vi "Check if string is integer.vi"(8 "error in (no error)":errorcluster, 11 "string in":string) -> (0 "error out":errorcluster, 2 "T = string contains an integer":bool, 3 "string out (duplicate)":string)   [LabVIEW 2021, in "Numeric Utilities.lvlib"]
uses:
  Numeric Utilities.lvlib
panel:
  # "Development\ncontrols/indicators useful for development and testing, but which are not outputs of the VI"
  # "Input\nInputs to the VI"
  # "Output\nOutputs of the VI"
  # "Description\n\nBlank VI with error handling case. \n\nSummarize the use of this VI in this space."
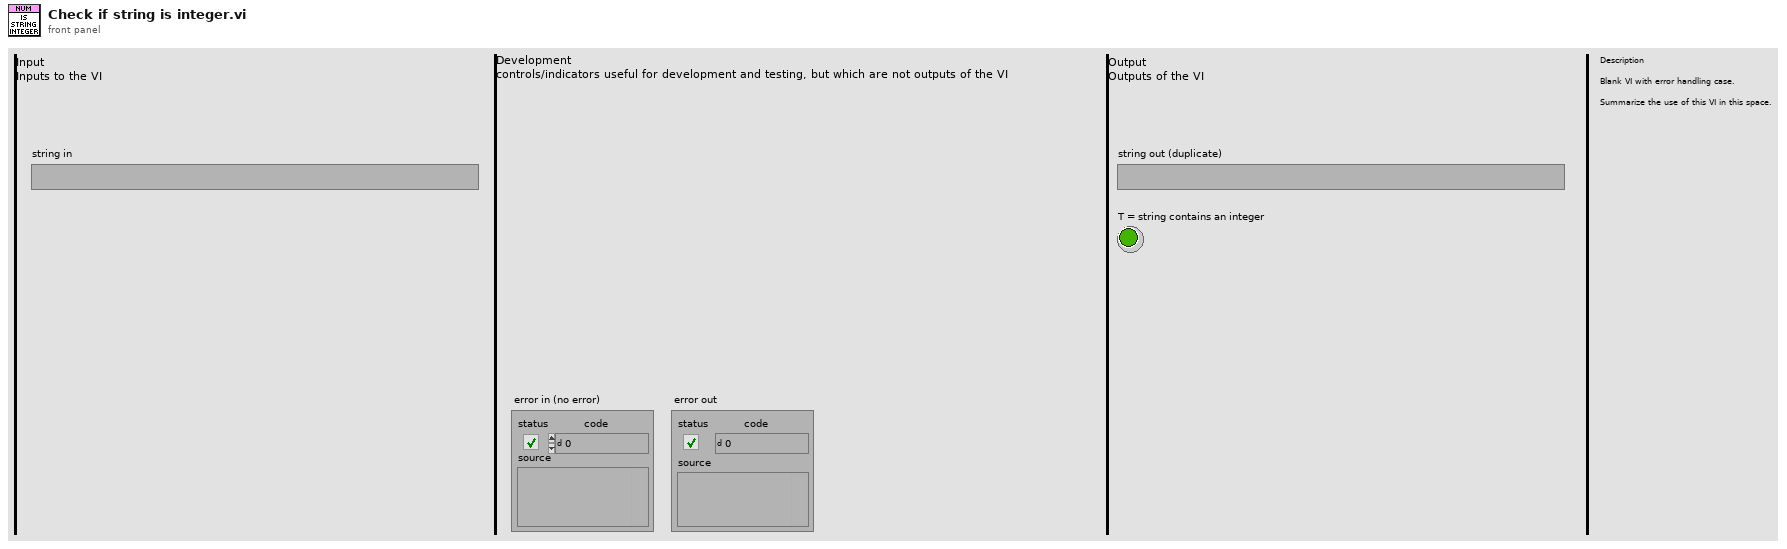
[diagram p1: front panel]
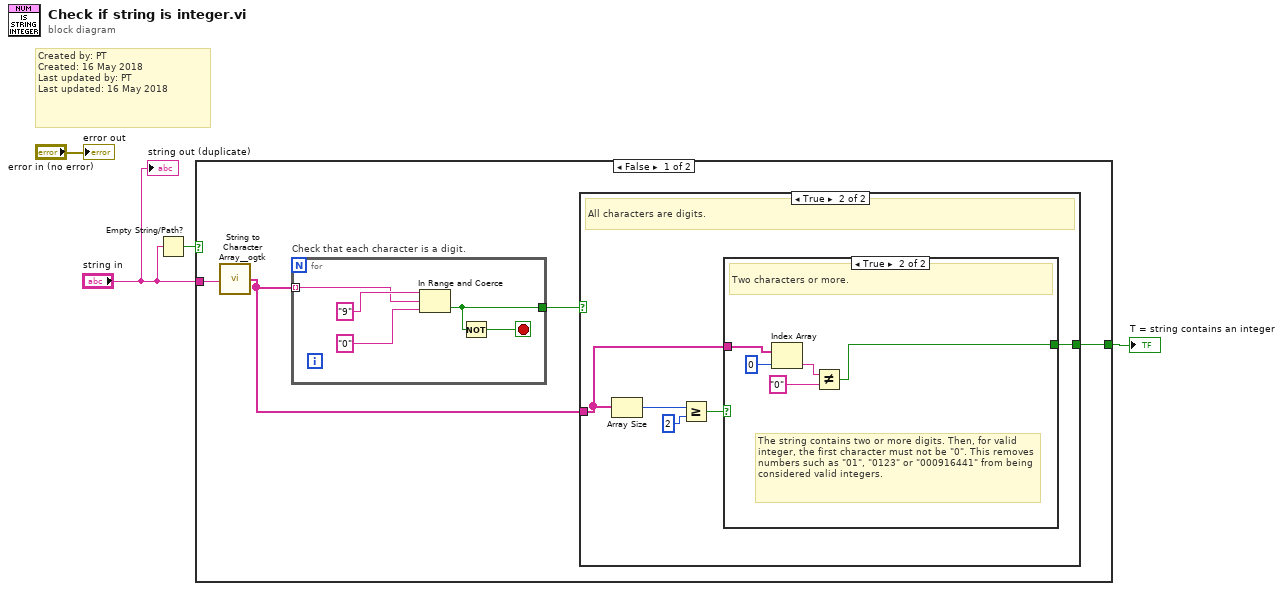
[diagram p0: block diagram]
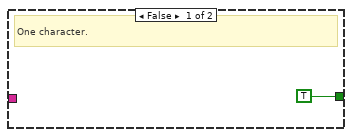
[diagram p3: hidden frame]
diagram:
  # "Created by: PT\nCreated: 16 May 2018\nLast updated by: PT\nLast updated: 16 May 2018"
  n1 = Empty String/Path?(string/path="string in") -> (empty?=w2:bool)
  n2 = case shown="False" w2 {
    tunnel: "string in" -> [w8 _]
    tunnel: [w5 _] -> w1
    frame False {
      n3 = call <userlib>:"String to Character Array__ogtk.vi"("Input String"=w8) -> ("Character Array"=w6:string[])
      n4 = for "Check that each character is a digit." {
        tunnel: w6 -> [w22] mode=indexing
        tunnel: [w20] -> w7
        stop <- w21 stop-if-true
        n5 = In Range and Coerce(upper limit="9", x=w22, lower limit="0") -> (In Range?=w20:bool)  [unwired: 1 out]
        n6 = Not(x=w20) -> (.not. x?=w21:bool)
      }
      n7 = case shown="True" w7 {
        tunnel: w6 -> [_ w9]
        tunnel: [_ w10] -> w5
        frame False {
          # "Some characters are NOT digits."
        }
        frame True {
          # "All characters are digits."
          n8 = Array Size(array=w9) -> (size(s)=w13:i32)
          n9 = Greater Or Equal?(x=w13, y=2) -> (x >= y?=w11:bool)
          n10 = case shown="True" w11 {
            tunnel: [TRUE w15] -> w10
            tunnel: w9 -> [_ w19]
            frame False {
              # "One character."
            }
            frame True {
              # "The string contains two or more digits. Then, for valid integer, the first character must not be \"0\". This removes numbers such as \"01\", \"0123\" or \"000916441\" from being considered valid integers."
              # "Two characters or more."
              n11 = Index Array(array=w19, index=0) -> (element=w17:string)
              n12 = Not Equal?(x=w17, y="0") -> (x != y?=w15:bool)
            }
          }
        }
      }
    }
    frame True {
    }
  }
  "T = string contains an integer" <- w1
  "error out" <- "error in (no error)"
  "string out (duplicate)" <- "string in"
